vi "shutdown_computer.vi"   [LabVIEW 2017]
doc: "This vi when run will shut down the computer and close labview for you. The VI will work with LabVIEW 6.1 or higher and a Windows XP machine."
panel:
  # "This vi when run will shut down the computer and close labview for you.  \nThe VI will work with LabVIEW 6.1 or higher and a Windows XP machine."
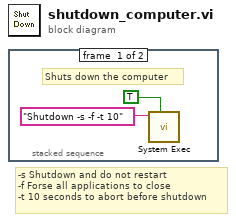
[diagram p0: block diagram]
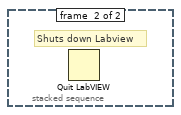
[diagram p2: hidden frame]
diagram:
  # "-s Shutdown and do not restart\n-f Forse all applications to close\n-t 10 seconds to abort before shutdown"
  n1 = stacked-sequence {
    frame #0 {
      # "Shuts down the computer"
      n2 = call <vilib>:"System Exec.vi"("wait until completion? (T)"=TRUE, "command line"="Shutdown -s -f -t 10") -> ()  [unwired: 6 in, 4 out]
    }
    frame #1 {
      # "Shuts down Labview"
      n3 = Quit LabVIEW() -> ()  [unwired: 1 in]
    }
  }
